vi "Merge.vi"(9 "new message":refnum<class "Channel Message.lvclass">, 11 "already enqueued message":refnum<class "Gesture Wrapper.lvclass">) -> (1 "merged?":bool, 3 "merged message":refnum<class "Gesture Wrapper.lvclass">)   [LabVIEW 2023, in "Gesture Wrapper.lvclass"]
doc: "Merge the gestures within two messages."
uses:
  Gesture Wrapper.lvclass
  <vilib>/ChannelSupport/Channel Message/Channel Message.lvclass
  Gesture Wrapper.lvclass/Gesture Wrapper.ctl
  Gesture/Gesture.lvclass
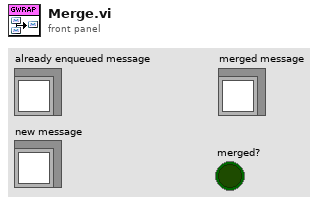
[diagram p1: front panel]
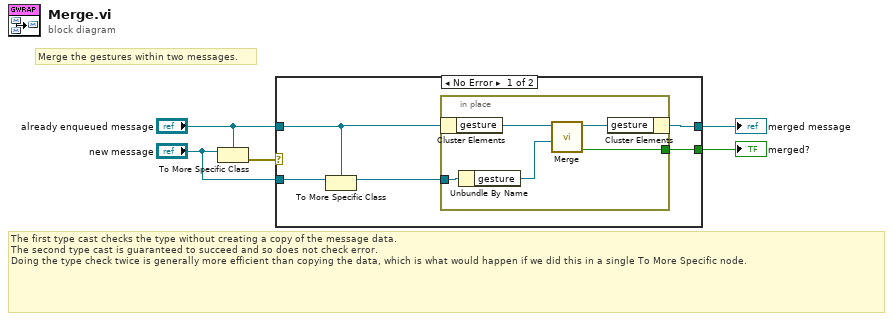
[diagram p0: block diagram]
diagram:
  # "Merge the gestures within two messages."
  # "The first type cast checks the type without creating a copy of the message data. \nThe second type cast is guaranteed to succeed and so does not check error. \nDoing the type check twice is generally more efficient than copying the data, which is what would happen if we did this in a single To More Specific node."
  n1 = To More Specific Class(target class="already enqueued message", reference="new message") -> (error out=w5:errorcluster)  [unwired: 1 in, 1 out]
  n2 = case shown="No Error" w5 {
    tunnel: "already enqueued message" -> [w8 w16]
    tunnel: [w10 w16] -> w3
    tunnel: [w9 _] -> w2
    tunnel: "new message" -> [w7 _]
    frame No Error {
      n3 = To More Specific Class(target class=w8, reference=w7) -> (specific class reference=w6:refnum<class "Gesture Wrapper.lvclass">)  [unwired: 1 in, 1 out]
      n4 = in-place {
        in-place-border: w6 -> [w13]
        in-place-border: [w11] -> w9
        n5 = in-place-cluster #1(w8) -> ("gesture"=w15:refnum<class "Gesture.lvclass">)
        n6 = Unbundle By Name(w13) -> ("gesture"=w12:refnum<class "Gesture.lvclass">)
        n7 = call-dynamic "Merge.vi"("new gesture in"=w12, "gesture in"=w15) -> ("merged?"=w11:bool, "gesture out"=w14:refnum<class "Gesture.lvclass">)  [unwired: 8 in]
        n8 = in-place-cluster #1("gesture"=w14) -> (w10:refnum<class "Gesture Wrapper.lvclass">)
      }
    }
    frame Error {
    }
  }
  "merged message" <- w3
  "merged?" <- w2
